vi "SeCrTs-AI V Start .vi"(8 "error in":errorcluster, 9 "AI V":T1(array[cluster]), 11 "Refnum in":refnum<k21>) -> (0 "error out":errorcluster, 3 "Refnum out":refnum<k21>)   [LabVIEW 2022 SP3]
doc: "This VI is for start for Analog voltage Start task"
uses:
  <vilib>/DAQmx/configure/timing.llb/DAQmx Timing (Sample Clock).vi
  <vilib>/DAQmx/configure/trigger.llb/DAQmx Start Trigger (Digital Edge).vi
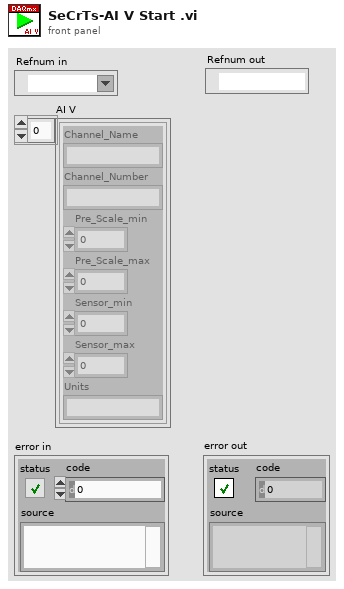
[diagram p1: front panel]
types:
  T1 = cluster{"Channel_Name":string, "Channel_Number":string, "Pre_Scale_min":dbl, "Pre_Scale_max":dbl, "Sensor_min":dbl, "Sensor_max":dbl, "Units":string}[]
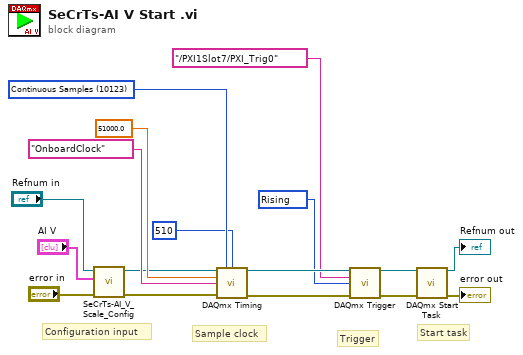
[diagram p0: block diagram]
diagram:
  w12 = 10280 items=["Rising"=10280, "Falling"=10171] ("edge")
  w9 = 10123 items=["Finite Samples"=10178, "Continuous Samples"=10123, "Hardware Timed Single Point"=12522] ("sample mode")
  # "Start task"
  # "Trigger"
  # "Sample clock"
  # "Configuration input"
  n1 = call "SeCrTs-AI_V_Scale_Config.vi"("error in"="error in", "AI C"="AI V", "task in"="Refnum in") -> ("error out"=w1:errorcluster, "task out"=w7:refnum<k21>)  [unwired: 7 in]
  n2 = call-poly <vilib>:"DAQmx Timing.vi"("task/channels in"=w7, "sample mode"=w9, "samples per channel"=510, "rate"=51000.0, "source"=tag "OnboardClock", "error in"=w1) -> ("task out"=w14:refnum<k21>, "error out"=w4:errorcluster)  [unwired: 8 in]
  n3 = call-poly <vilib>:"DAQmx Trigger.vi"("task/channels in"=w14, "source"=tag "/PXI1Slot7/PXI_Trig0", "edge"=w12, "error in"=w4) -> ("task out"=w16:refnum<k21>, "error out"=w15:errorcluster)  [unwired: 10 in]
  n4 = call <vilib>:"DAQmx Start Task.vi"("task/channels in"=w16, "error in"=w15) -> ("task out"=→"Refnum out":refnum<k21>, "error out"=→"error out":errorcluster)  [unwired: 12 in]
